vi "La_Calc.vi"() -> ()   [LabVIEW 2019]
uses:
  <vilib>/gmath/SpecialFunctions.llb/Gamma Function.vi
  <vilib>/regexp/Match Regular Expression.xnode
  <vilib>/gmath/NI_Gmath.lvlib
panel:
  out "Bandera\nde Ans":bool
  out "Del":bool
  out "result string":string
  in  "Ans":ext
  in  "Boton .":bool
  in  "Boton nqrt":bool
  in  "Boton sqrt":bool
  in  "Boton e":bool
  in  "Boton )":bool
  in  "Boton (":bool
  in  "boton asen":bool
  in  "Boton crt":bool
  in  "Boton tan(x)":bool
  in  "Boton cos(x)":bool
  in  "Boton sen(x)":bool caption="1"
  in  "Boton tanh":bool
  in  "Boton cosh":bool
  in  "Boton sech":bool caption="1"
  in  "Boton /":bool
  in  "Boton *":bool
  in  "Boton -":bool
  in  "Boton =":bool
  in  "Boton Pi":bool
  in  "Boton +":bool
  in  "Boton atan":bool
  in  "Boton acos":bool
  in  "Boton R2D":bool
  in  "Boton D2R":bool
  in  "Boton Ans":bool
  out "Pantalla":string
  in  "Boton Log(x)":bool
  in  "Boton Ln":bool
  in  "Boton Log":bool caption="1"
  in  "Boton x^y":bool
  in  "Boton x^3":bool
  in  "Boton x^2":bool caption="1"
  in  "Boton x^-1":bool
  in  "Boton e^x":bool
  in  "Boton x!":bool caption="1"
  in  "Boton 0":bool
  in  "Boton DEL":bool
  in  "Boton C":bool
  in  "Boton 9":bool
  in  "Boton 8":bool
  in  "Boton 7":bool
  in  "Boton 6":bool
  in  "Boton 5":bool
  in  "Boton 4":bool
  in  "Boton 3":bool
  in  "Boton 2":bool
  in  "Boton 1":bool caption="1"
  # "La pantalla permite colocar cualquier cadena siempre y la evaluara si es evaluable.\nUse sintaxis de calculadora NO NATURAL."
  # "No se permite factoriales anidados.\nPero si se permiten varios factoriales tal que asi: 5!+3!+2!"
  # "Este es logaritmo base n, su sintaxis es la siguiente\nLOG20(300) calcula el logaritmo base 20 de 300\nLa base por sintaxis debe de ser un numero(puede\nser decimal o entero). No puede ser una operacion.\nY la base no debe de ir entre parentesis"
  # "En cuanto a los problemas de la\nfuncion LOG base n hay que decir\nque el bloque \"Match Regular \nExpression\" no funciona correctamente\nprobar la expresion regular\nLOG\\d(.*?)\\( y LOG(.*?)\\( y dan\ncon el bloque resultados\niguales, cualquier duda con las\nexpresiones regulares utilizadas\nhacermelo saber."
  # "Use coma en vez de punto.\nEsto por simplicidad, ya que la\nfuncion evular string usa comas\ny no puntos."
  # "C resetea la pantalla y el valor de Ans.\nR2D  es Radianes a grados.\nD2R es grados a radianes."
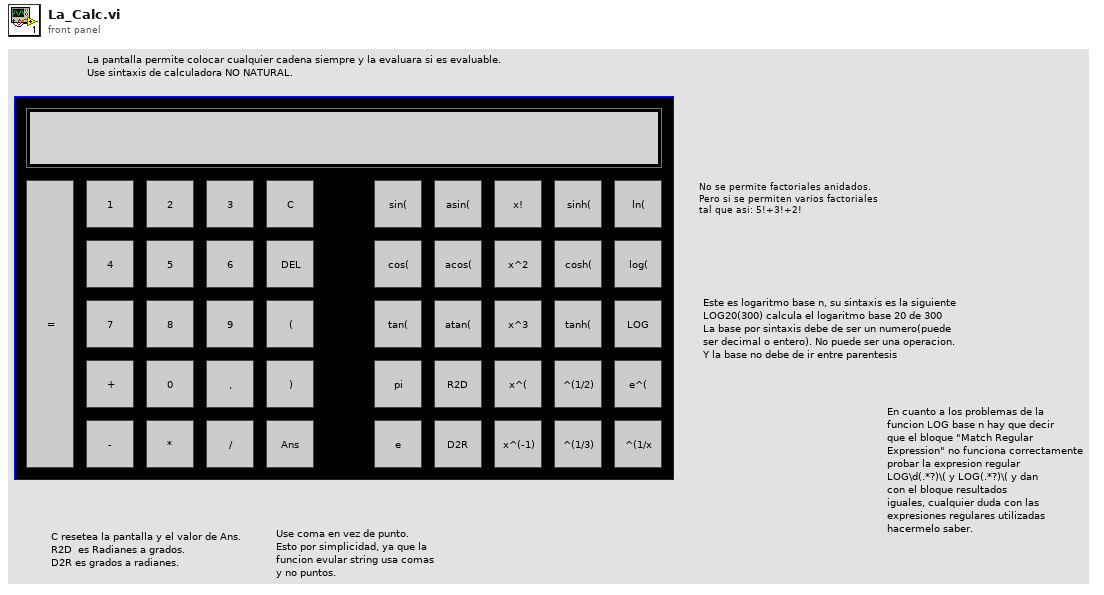
[diagram p1: front panel]
types:
  T1 = typedef "eventvkey.ctl" = enum16{"ASCII", "Enter", "Return", "Shift", "Ctrl", "Alt", "Cmd", "Opt", "Caps", "NumLock", "Clear", "Break", "Up", "Down", "Left", "Right", "Insert", "Delete", "Home", "End", "PageUp", "PageDown", "Escape", "Help", "Pause", "ScrollLock", "F1", "F2", "F3", "F4", "F5", "F6", "F7", "F8", "F9", "F10", "F11", "F12", "F13", "F14", "F15", "F16", "F17", "F18", "F19", "F20", "F21", "F22", "F23", "F24", "Play", "VolumeUp", "VolumeDown", "Mute", "Two Byte Char"}
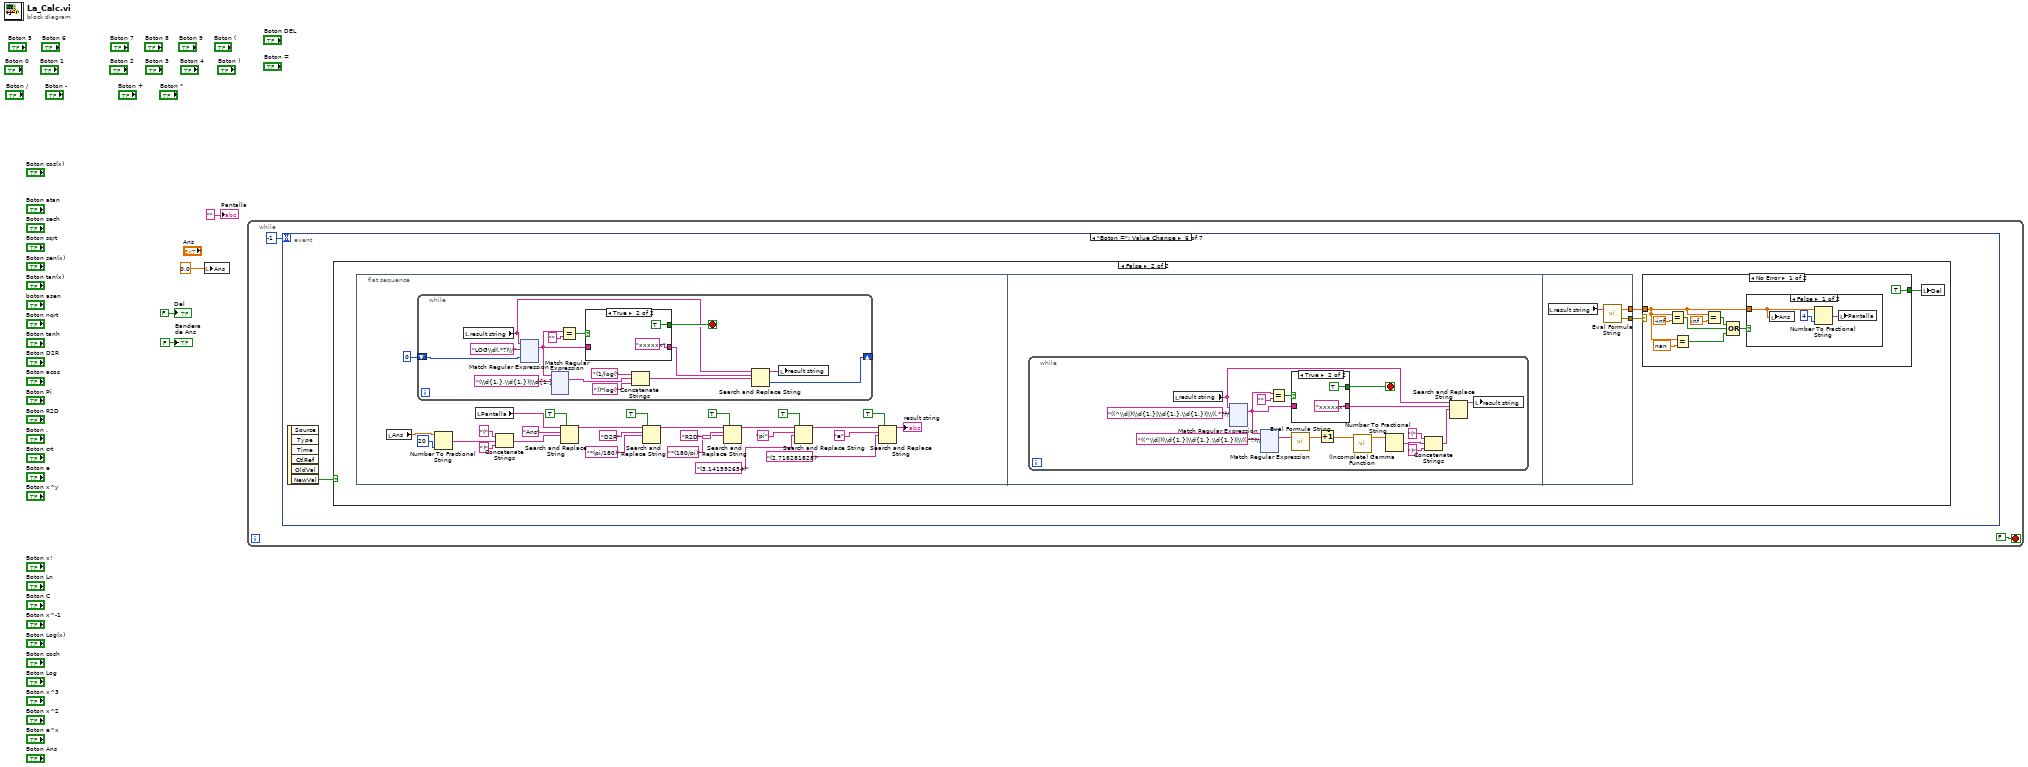
[diagram p0: block diagram]
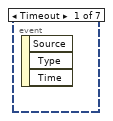
[diagram p2: hidden frame]
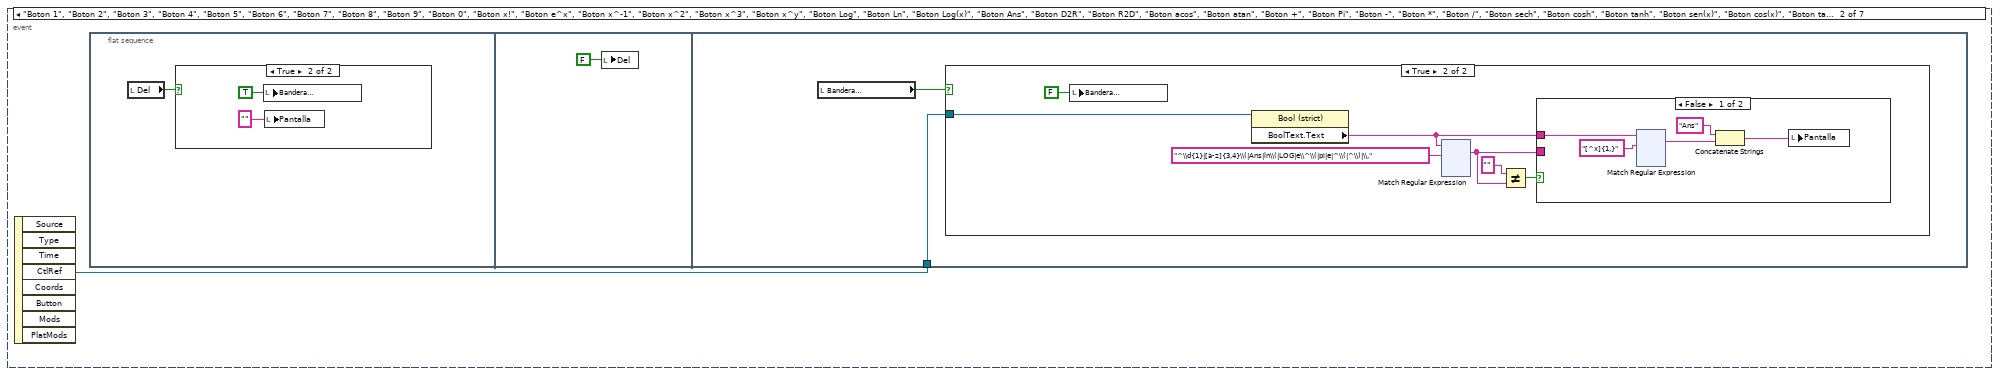
[diagram p3: hidden frame]
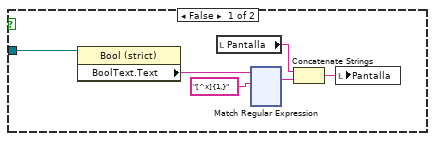
[diagram p5: hidden frame]
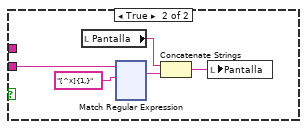
[diagram p6: hidden frame]
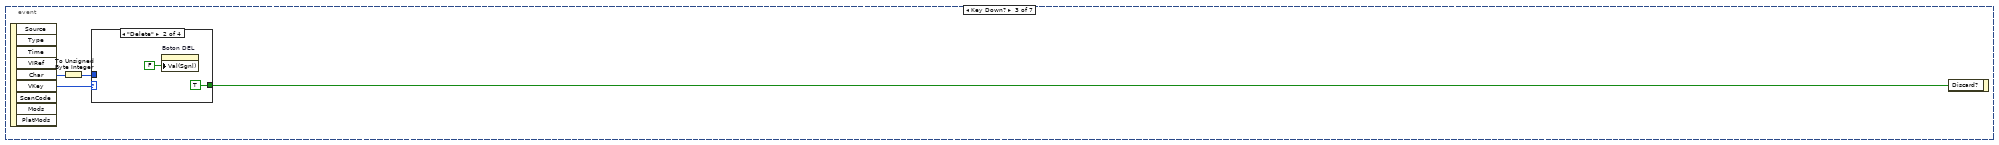
[diagram p7: hidden frame]
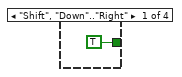
[diagram p8: hidden frame]
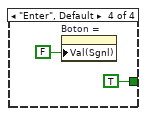
[diagram p10: hidden frame]
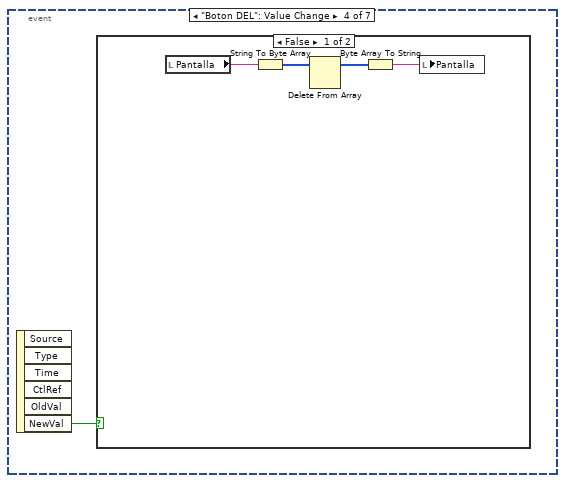
[diagram p11: hidden frame]
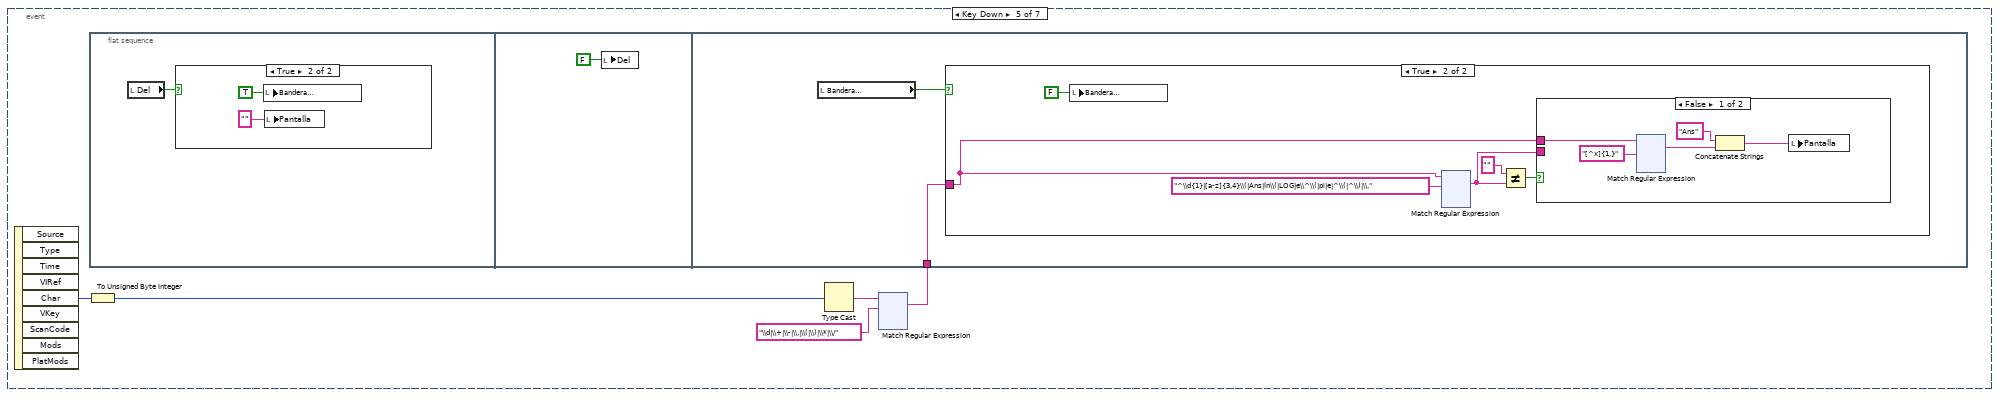
[diagram p13: hidden frame]
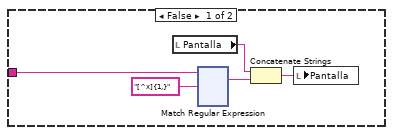
[diagram p15: hidden frame]
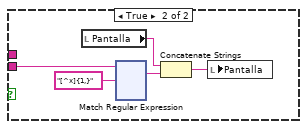
[diagram p16: hidden frame]
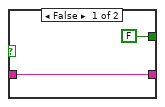
[diagram p18: hidden frame]
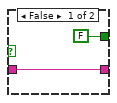
[diagram p19: hidden frame]
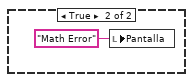
[diagram p20: hidden frame]
diagram:
  n1 = local write "Ans"(0.0) -> ()
  n2 = while {
    stop <- FALSE stop-if-true
    n3 = event shown="[5] \"Boton =\": Value Change" {
      selector: _ -> [_ _ _ _ _ _ _]
      dyn-events: _ -> [_ _ _ _ _ _ _]
      timeout: -1 -> [_ _ _ _ _ _ _]
      event Timeout {
        n4 = event-data() -> ()  [unwired: 1 in, 3 out]
      }
      event "Boton 1", "Boton 2", "Boton 3", "Boton 4", "Boton 5", "Boton 6", "Boton 7", "Boton 8", "Boton 9", "Boton 0", "Boton x!", "Boton e^x", "Boton x^-1", "Boton x^2", "Boton x^3", "Boton x^y", "Boton Log", "Boton Ln", "Boton Log(x)", "Boton Ans", "Boton D2R", "Boton R2D", "Boton acos", "Boton atan", "Boton +", "Boton Pi", "Boton -", "Boton *", "Boton /", "Boton sech", "Boton cosh", "Boton tanh", "Boton sen(x)", "Boton cos(x)", "Boton tan(x)", "Boton crt", "boton asen", "Boton (", "Boton )", "Boton e", "Boton sqrt", "Boton nqrt", "Boton .": Mouse Down {
        n5 = event-data() -> ("CtlRef"=w7:refnum<vi>)  [unwired: 1 in, 7 out]
        n6 = flat-sequence {
          tunnel: w7 -> [w12]
          frame #0 {
            n7 = local read "Del"() -> (w8:bool)
            n8 = case shown="True" w8 {
              frame False {
              }
              frame True {
                n9 = local write "Bandera\nde Ans"(TRUE ("Boolean")) -> ()
                n10 = local write "Pantalla"("" ("Pantalla")) -> ()
              }
            }
          }
          frame #1 {
            n11 = local write "Del"(FALSE ("Del")) -> ()
          }
          frame #2 {
            n12 = local read "Bandera\nde Ans"() -> (w13:bool)
            n13 = case shown="True" w13 {
              tunnel: w12 -> [w14 w140]
              frame False {
                n14 = property class="Bool (strict)"(reference=w14) -> ("BoolText.Text"=w18:string)  [unwired: 1 in, 2 out]
                n15 = local read "Pantalla"() -> (w19:string)
                n16 = xnode "Match Regular Expression"("input string"=w18, "regular expression"="[^x]{1,}") -> ("whole match"=w17:string)  [unwired: 4 in, 4 out]
                n17 = Concatenate Strings(w19, w17) -> (w16:string)
                n18 = local write "Pantalla"(w16) -> ()
              }
              frame True {
                n19 = local write "Bandera\nde Ans"(FALSE ("Boolean")) -> ()
                n20 = property class="Bool (strict)"(reference=w140) -> ("BoolText.Text"=w135:string)  [unwired: 1 in, 2 out]
                n21 = xnode "Match Regular Expression"("input string"=w135, "regular expression"="^\\d{1}|[a-z]{3,4}\\(|Ans|ln\\(|LOG|e\\^\\(|pi|e|^\\(|^\\)|\\,") -> ("whole match"=w136:string)  [unwired: 4 in, 4 out]
                n22 = Not Equal?(x="", y=w136) -> (x != y?=w137:bool)
                n23 = case shown="False" w137 {
                  tunnel: w136 -> [_ w260]
                  tunnel: w135 -> [w142 _]
                  frame False {
                    n24 = xnode "Match Regular Expression"("input string"=w142, "regular expression"="[^x]{1,}") -> ("whole match"=w144:string)  [unwired: 4 in, 4 out]
                    n25 = Concatenate Strings("Ans" ("string"), w144) -> (w145:string)
                    n26 = local write "Pantalla"(w145) -> ()
                  }
                  frame True {
                    n27 = local read "Pantalla"() -> (w264:string)
                    n28 = xnode "Match Regular Expression"("input string"=w260, "regular expression"="[^x]{1,}") -> ("whole match"=w263:string)  [unwired: 4 in, 4 out]
                    n29 = Concatenate Strings(w264, w263) -> (w262:string)
                    n30 = local write "Pantalla"(w262) -> ()
                  }
                }
              }
            }
          }
        }
      }
      event Key Down? {
        n31 = event-data() -> ("Char"=w496:i16, "VKey"=w495:T1)  [unwired: 1 in, 7 out]
        n32 = To Unsigned Byte Integer(number=w496) -> (unsigned 8bit integer=w494:u8)
        n33 = case shown="\"Delete\"" w495 {
          tunnel: w494 -> [_ _ _ _]
          tunnel: [TRUE ("Value (Signaling)") TRUE ("Value (Signaling)") _ TRUE ("Value (Signaling)")] -> w493
          frame "Shift", "Down".."Right" {
          }
          frame "Delete" {
            n34 = property on="Boton DEL" class="Bool (strict)"("Val(Sgnl)"=FALSE ("Value (Signaling)")) -> ()  [unwired: 2 in, 2 out]
          }
          frame "ASCII" {
          }
          frame "Enter", Default {
            n35 = property on="Boton =" class="Bool (strict)"("Val(Sgnl)"=FALSE ("Value (Signaling)")) -> ()  [unwired: 2 in, 2 out]
          }
        }
        n36 = event-data("Discard?"=w493) -> ()  [unwired: 1 in, 1 out]
      }
      event "Boton DEL": Value Change {
        n37 = event-data() -> ("NewVal"=w502:bool)  [unwired: 1 in, 5 out]
        n38 = case shown="False" w502 {
          frame False {
            n39 = local read "Pantalla"() -> (w505:string)
            n40 = String To Byte Array(string=w505) -> (unsigned byte array=w506:u8[])
            n41 = Delete From Array(array=w506) -> (array with subset deleted=w504:u8[])  [unwired: 2 in, 1 out]
            n42 = Byte Array To String(unsigned byte array=w504) -> (string=w503:string)
            n43 = local write "Pantalla"(w503) -> ()
          }
          frame True {
          }
        }
      }
      event Key Down {
        n44 = event-data() -> ("Char"=w510:i16)  [unwired: 1 in, 8 out]
        n45 = To Unsigned Byte Integer(number=w510) -> (unsigned 8bit integer=w511:u8)
        n46 = flat-sequence {
          tunnel: w507 -> [w516]
          frame #0 {
            n47 = local read "Del"() -> (w512:bool)
            n48 = case shown="True" w512 {
              frame False {
              }
              frame True {
                n49 = local write "Bandera\nde Ans"(TRUE ("Boolean")) -> ()
                n50 = local write "Pantalla"("" ("Pantalla")) -> ()
              }
            }
          }
          frame #1 {
            n51 = local write "Del"(FALSE ("Del")) -> ()
          }
          frame #2 {
            n52 = local read "Bandera\nde Ans"() -> (w517:bool)
            n53 = case shown="True" w517 {
              tunnel: w516 -> [w518 w637]
              frame False {
                n54 = local read "Pantalla"() -> (w522:string)
                n55 = xnode "Match Regular Expression"("input string"=w518, "regular expression"="[^x]{1,}") -> ("whole match"=w521:string)  [unwired: 4 in, 4 out]
                n56 = Concatenate Strings(w522, w521) -> (w520:string)
                n57 = local write "Pantalla"(w520) -> ()
              }
              frame True {
                n58 = local write "Bandera\nde Ans"(FALSE ("Boolean")) -> ()
                n59 = xnode "Match Regular Expression"("input string"=w637, "regular expression"="^\\d{1}|[a-z]{3,4}\\(|Ans|ln\\(|LOG|e\\^\\(|pi|e|^\\(|^\\)|\\,") -> ("whole match"=w639:string)  [unwired: 4 in, 4 out]
                n60 = Not Equal?(x="", y=w639) -> (x != y?=w640:bool)
                n61 = case shown="False" w640 {
                  tunnel: w639 -> [_ w762]
                  tunnel: w637 -> [w644 _]
                  frame False {
                    n62 = xnode "Match Regular Expression"("input string"=w644, "regular expression"="[^x]{1,}") -> ("whole match"=w646:string)  [unwired: 4 in, 4 out]
                    n63 = Concatenate Strings("Ans" ("string"), w646) -> (w647:string)
                    n64 = local write "Pantalla"(w647) -> ()
                  }
                  frame True {
                    n65 = local read "Pantalla"() -> (w766:string)
                    n66 = xnode "Match Regular Expression"("input string"=w762, "regular expression"="[^x]{1,}") -> ("whole match"=w765:string)  [unwired: 4 in, 4 out]
                    n67 = Concatenate Strings(w766, w765) -> (w764:string)
                    n68 = local write "Pantalla"(w764) -> ()
                  }
                }
              }
            }
          }
        }
        n69 = Type Cast(x=w511) -> (*(type *) &x=w508:string)  [unwired: 1 in]
        n70 = xnode "Match Regular Expression"("input string"=w508, "regular expression"="\\d|\\+|\\-|\\,|\\(|\\)|\\*|\\/") -> ("whole match"=w507:string)  [unwired: 4 in, 4 out]
      }
      event "Boton =": Value Change {
        n71 = event-data() -> ("NewVal"=w1109:bool)  [unwired: 1 in, 5 out]
        n72 = case shown="False" w1109 {
          frame True {
          }
          frame False {
            n73 = flat-sequence {
              tunnel: [w1638] -> w1112
              tunnel: [w1637] -> w1111
              frame #0 {
                n74 = local read "Ans"() -> (w1119:ext)
                n75 = while {
                  shift-right: [w1149] -> _
                  shift-left: 0 ("offset past match") -> [w1148]
                  stop <- w1145 stop-if-true
                  n76 = local read "result string"() -> (w1143:string)
                  n77 = xnode "Match Regular Expression"("input string"=w1143, "regular expression"="LOG\\d(.*?)\\(", "offset (0)"=w1148) -> ("whole match"=w1142:string)  [unwired: 3 in, 4 out]
                  n78 = xnode "Match Regular Expression"("input string"=w1142, "regular expression"="(\\d{1,},\\d{1,})|\\d{1,}") -> ("whole match"=w1151:string)  [unwired: 4 in, 4 out]
                  n79 = Equal?(x=w1142, y="") -> (x = y?=w1147:bool)
                  n80 = case shown="True" w1147 {
                    tunnel: [FALSE TRUE] -> w1145
                    tunnel: w1142 -> [w1384 _]
                    tunnel: [w1384 "xxxxxx" ("before match")] -> w1144
                    frame False {
                    }
                    frame True {
                    }
                  }
                  n81 = Concatenate Strings("(1/log(" ("string"), w1151, "))*log(" ("string")) -> (w1141:string)
                  n82 = Search and Replace String(input string=w1143, search string=w1144, replace string=w1141) -> (result string=w1150:string, offset past replacement=w1149:i32)  [unwired: 5 in, 2 out]
                  n83 = local write "result string"(w1150) -> ()
                }
                n84 = Number To Fractional String(number=w1119, precision (6)=i16 20) -> (F-format string=w1115:string)  [unwired: 2 in]
                n85 = local read "Pantalla"() -> (w1122:string)
                n86 = Concatenate Strings("(" ("string"), w1115, ")" ("string")) -> (w1114:string)
                n87 = Search and Replace String(replace all?=TRUE ("replace all? (F)"), input string=w1122, search string="Ans", replace string=w1114) -> (result string=w1121:string)  [unwired: 4 in, 3 out]
                n88 = Search and Replace String(replace all?=TRUE ("replace all? (F)"), input string=w1121, search string="D2R", replace string="*(pi/180)" ("replace string (\"\")")) -> (result string=w1126:string)  [unwired: 4 in, 3 out]
                n89 = Search and Replace String(replace all?=TRUE ("replace all? (F)"), input string=w1126, search string="R2D", replace string="*(180/pi)" ("replace string (\"\")")) -> (result string=w1125:string)  [unwired: 4 in, 3 out]
                n90 = Search and Replace String(replace all?=TRUE ("replace all? (F)"), input string=w1125, search string="pi", replace string="(3,141592654)" ("replace string (\"\")")) -> (result string=w1139:string)  [unwired: 4 in, 3 out]
                n91 = Search and Replace String(replace all?=TRUE ("replace all? (F)"), input string=w1139, search string="e", replace string="(2,718281828)" ("replace string (\"\")")) -> (result string=→"result string":string)  [unwired: 4 in, 3 out]
              }
              frame #1 {
                n92 = while {
                  stop <- w1397 stop-if-true
                  n93 = local read "result string"() -> (w1403:string)
                  n94 = xnode "Match Regular Expression"("input string"=w1403, "regular expression"="((^\\d|)(\\d{1,}|\\d{1,},\\d{1,})|\\((.*?)\\))\\!") -> ("whole match"=w1396:string)  [unwired: 4 in, 4 out]
                  n95 = xnode "Match Regular Expression"("input string"=w1396, "regular expression"="((^\\d|)(\\d{1,}|\\d{1,},\\d{1,})|\\((.*?)\\))") -> ("whole match"=w1402:string)  [unwired: 4 in, 4 out]
                  n96 = Equal?(x=w1396, y="") -> (x = y?=w1398:bool)
                  n97 = case shown="True" w1398 {
                    tunnel: [FALSE TRUE] -> w1397
                    tunnel: w1396 -> [w1405 _]
                    tunnel: [w1405 "xxxxxx" ("before match")] -> w1395
                    frame False {
                    }
                    frame True {
                    }
                  }
                  n98 = call <vilib>:"Eval Formula String.vi"("formula"=w1402) -> ("y value"=w1389:dbl)  [unwired: 1 in, 1 out]
                  n99 = Increment(x=w1389) -> (x+1=w1388:dbl)
                  n100 = call-poly <vilib>:"(Incomplete) Gamma Function.vi"("x"=w1388) -> ("g(x)"=w1387:dbl)  [unwired: 10 in]
                  n101 = Number To Fractional String(number=w1387) -> (F-format string=w1393:string)  [unwired: 3 in]
                  n102 = Concatenate Strings("(" ("string"), w1393, ")" ("string")) -> (w1392:string)
                  n103 = Search and Replace String(input string=w1403, search string=w1395, replace string=w1392) -> (result string=w1394:string)  [unwired: 5 in, 3 out]
                  n104 = local write "result string"(w1394) -> ()
                }
              }
              frame #2 {
                n105 = local read "result string"() -> (w1636:string)
                n106 = call <vilib>:"Eval Formula String.vi"("formula"=w1636) -> ("error out"=w1638:errorcluster, "y value"=w1637:dbl)  [unwired: 1 in]
              }
            }
            n107 = case shown="No Error" w1112 {
              tunnel: w1111 -> [w1639 _]
              tunnel: [TRUE TRUE] -> w1110
              frame No Error {
                n108 = Equal?(x=w1639, y=-inf) -> (x = y?=w1645:bool)
                n109 = Equal?(x=w1639, y=nan) -> (x = y?=w1646:bool)
                n110 = Equal?(x=w1639, y=inf) -> (x = y?=w1644:bool)
                n111 = Compound Arithmetic op=OR(w1644, w1645, w1646) -> (w1640:bool)
                n112 = case shown="False" w1640 {
                  tunnel: w1639 -> [w1648 _]
                  frame False {
                    n113 = local write "Ans"(w1648) -> ()
                    n114 = Number To Fractional String(number=w1648, precision (6)=i16 4) -> (F-format string=w1650:string)  [unwired: 2 in]
                    n115 = local write "Pantalla"(w1650) -> ()
                  }
                  frame True {
                    n116 = local write "Pantalla"("Math Error") -> ()
                  }
                }
              }
              frame Error {
                n117 = local write "Pantalla"("SYNTAX ERROR" ("String")) -> ()
              }
            }
            n118 = local write "Del"(w1110) -> ()
          }
        }
      }
      event "Boton C": Mouse Down {
        n119 = event-data() -> ()  [unwired: 1 in, 8 out]
        n120 = local write "Ans"(0.0 ("Ans")) -> ()
        n121 = local write "Pantalla"("" ("Pantalla")) -> ()
      }
    }
  }
  "Pantalla" <- "" ("String")
  "Del" <- FALSE ("Del")
  "Bandera\nde Ans" <- FALSE ("Boolean")
